vi "Path Relative to Root.vi"(10 "ItemPath":path, 11 "RootDir":path) -> (3 "ItemPath (Relative to Root)":path)   [LabVIEW 2013, in "SET Project Editor.lvlib"]
doc: "Path Relative to Root.vi\n\nBuild the path of a file relative to a root directory.\n\nInputs\nItemPath: Absolute path to file\nRootDir: Absolute path to the root directory.\n\nOutput\nItemPath (Relative to Root): Relative path to file."
uses:
  SET Project Editor.lvlib
panel:
  # "Path Relative to Root.vi\n\nBuild the path of a file relative to a root directory.\n\nInputs\nItemPath: Absolute path to file\nRootDir: Absolute path to the root directory.\n\nOutput\nItemPath (Relative to Root): Relative path to file."
  # "License: BSD (2-Clause) - http://opensource.org/licenses/BSD-2-Clause \n\nCopyright (c) 2014, Ryan Porter\nAll rights reserved."
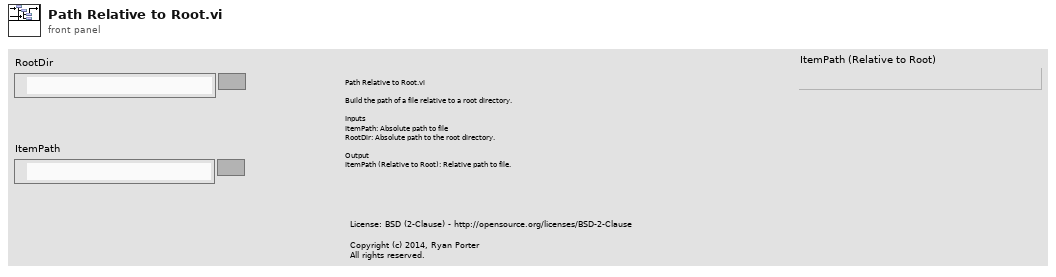
[diagram p1: front panel]
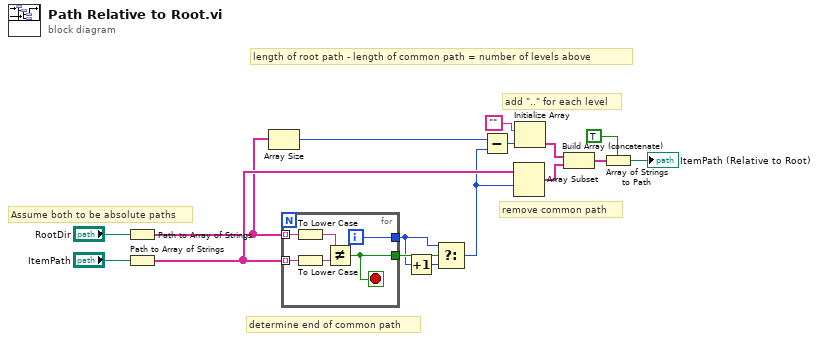
[diagram p0: block diagram]
diagram:
  # "length of root path - length of common path = number of levels above"
  # "add \"..\" for each level"
  # "remove common path"
  # "determine end of common path"
  # "Assume both to be absolute paths"
  n1 = Path to Array of Strings(0:"RootDir") -> (2:w9:string[])  [unwired: 1 out]
  n2 = Path to Array of Strings(0:"ItemPath") -> (2:w11:string[])  [unwired: 1 out]
  n3 = Array Size(array=w9) -> (size(s)=w10:i32)
  n4 = for {
    tunnel: w9 -> [w22] mode=indexing
    tunnel: w11 -> [w21] mode=indexing
    tunnel: [w18] -> w2
    tunnel: [w17] -> w4
    i -> [w18]
    stop <- w17 stop-if-true
    n5 = To Lower Case(string=w22) -> (all lower case string=w20:string)
    n6 = To Lower Case(string=w21) -> (all lower case string=w19:string)
    n7 = Not Equal?(x=w20, y=w19) -> (x != y?=w17:bool)
  }
  n8 = Increment(x=w2) -> (x+1=w3:i32)
  n9 = Select(t=w2, s=w4, f=w3) -> (s? t:f=w1:i32)
  n10 = Subtract(x=w10, y=w1) -> (x-y=w12:i32)
  n11 = Array Subset(array=w11, index=w1) -> (w14:string[])  [unwired: 1 in]
  n12 = Initialize Array("", w12) -> (w13:string[])
  n13 = Build Array (concatenate)(w13, w14) -> (w15:string[])
  n14 = Array of Strings to Path(0:w15, 1:TRUE ("relative")) -> (2:→"ItemPath (Relative to Root)":path)
